vi "DeQueueElement.vi"(8 "Error Array In":errorcluster[](array[cluster]), 11 "Queue In":refnum<queue>) -> (0 "Error Array Out":errorcluster[](array[cluster]), 1 "Data":variant, 2 "Message":string, 3 "Queue Out":refnum<queue>)   [LabVIEW 2018, in "Visualization.lvlib" / "VisualizeBase.lvclass"]
doc: "This VI extracts the message and data from the queue."
uses:
  VisualizeBase/VisualizeBase_class/VisualizeBase.lvclass
  Typedefs/MsgType.ctl
  <userlib>/NIST/NISTErrorLib/NISTErrorLib.lvlib
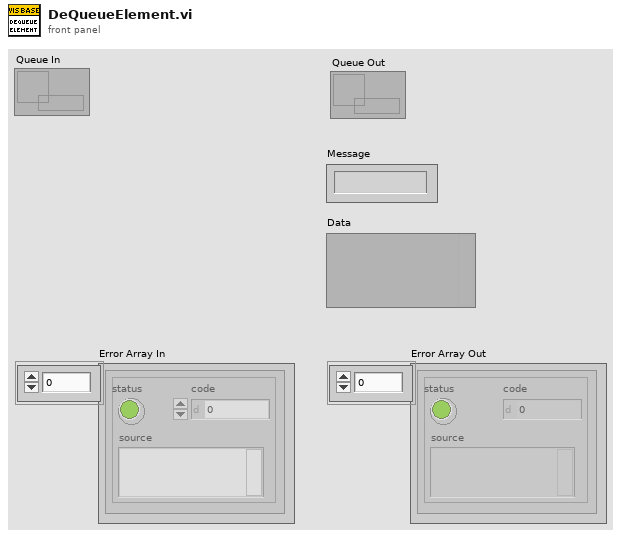
[diagram p1: front panel]
types:
  T1 = typedef "Visualization.lvlib/VisualizeBase.lvclass/MsgType.ctl" = cluster{"Message":string, "Data":variant}
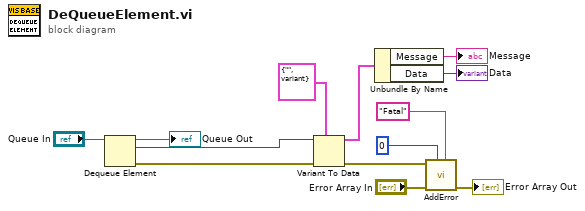
[diagram p0: block diagram]
diagram:
  n1 = Dequeue Element(queue="Queue In") -> (queue out=→"Queue Out":refnum<queue>, element=w13:variant, error out=w12:errorcluster)  [unwired: 2 in, 1 out]
  n2 = Variant To Data(error in=w12, type=T1 {"Message"="", "Data"=variant} ("clMsgType"), Variant=w13) -> (data=w10:T1, error out=w5:errorcluster)
  n3 = Unbundle By Name(w10) -> ("Message"=→"Message":string, "Data"=→"Data":variant)
  n4 = call <userlib>:"AddError.vi"("Severity"="Fatal" ("String"), "Priority"=u8 0, "ErrorArray In"="Error Array In", "error in (no error)"=w5) -> ("ErrorArray Out"=→"Error Array Out":errorcluster[])  [unwired: 6 in, 1 out]
